vi "Teleop.vi"(10 "Match Info":T1={"Autonomous Elapsed Seconds"=0.0, "TeleOp Elapsed Seconds"=0.0, "Disabled Elapsed Seconds"=0.0, "Visited Autonomous"=FALSE, "Visited TeleOp"=FALSE, "Visited Disabled"=FALSE, "Autonomous Settings"={"Autonomous Style"=enum."Independent", "VI Refnum"=refnum}}, 11 "Call Context":T2) -> ()   [LabVIEW 2012]
doc: "This VI is called for each TeleOp packet received from the DS where the robot is not disabled. It is often used to read from the joysticks and update I/O or to update setpoints for timed control loops. It should complete and return within 20 milliseconds or it may miss DS packets."
uses:
  <vilib>/Rock Robotics/WPI/DriverStation/WPI_DriverStationDerivedRobotMode.ctl
  <vilib>/Rock Robotics/WPI/DriverStation/WPI_DriverStationMatch Info.ctl
  RefnameEnum.ctl
  QueueEnum.ctl
  Robot Global Data.vi
  <vilib>/Rock Robotics/WPI/Joystick/WPI_JoystickGetSetRefNum.vi
  State_Machine_Enum.ctl
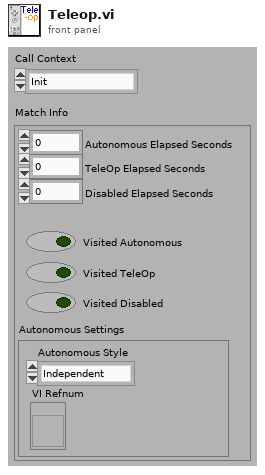
[diagram p1: front panel]
types:
  T1 = typedef "WPI_DriverStationMatch Info.ctl" = cluster{"Autonomous Elapsed Seconds":dbl, "TeleOp Elapsed Seconds":dbl, "Disabled Elapsed Seconds":dbl, "Visited Autonomous":bool, "Visited TeleOp":bool, "Visited Disabled":bool, "Autonomous Settings":cluster{"Autonomous Style":enum16{"Iterative", "Independent"}, "VI Refnum":refnum<vi>}}
  T2 = typedef "WPI_DriverStationDerivedRobotMode.ctl" = enum16{"Init", "Execute", "Stop"}
  T3 = typedef "State_Machine_Enum.ctl" = enum16{"Idle", "Start", "Do", "Stop", "Init"}
  T4 = typedef "QueueEnum.ctl" = enum16{"cTankDrive", "cClimb", "cLauncherAngle", "cLauncherWheel", "cFirePneumatic"}
  T5 = typedef "RefnameEnum.ctl" = enum16{"FireLauncher", "Climber", "Shield", "TankDrive", "DriveEncoderL", "DriveEncoderR", "LauncherMotorRPM", "LauncherEncoderAnalog", "LauncherEncoderRPM", "ShooterLS", "DriveAlignLSLeft", "DriveAlignLSRight", "ClimbingLS", "LauncherEncoderAngle", "LauncherMotorAngle", "Gamepad1", "Gamepad2", "Compressor", "ClimbWeightSol3", "ClimbWeightSol4"}
  T6 = typedef "WPI_JoystickDevRef.ctl" = cluster{"Device":T7}
  T7 = typedef "WPI_JoystickDeviceEnum.ctl" = enum16{"USB 1", "USB 2", "USB 3", "USB 4", "Kinect 1", "Kinect 2"}
  T8 = typedef "WPI_JoystickButtonState.ctl" = cluster{"Button 1":bool, "Button 2":bool, "Button 3":bool, "Button 4":bool, "Button 5":bool, "Button 6":bool, "Button 7":bool, "Button 8":bool, "Button 9":bool, "Button 10":bool, "Button 11":bool, "Button 12":bool}
  T9 = cluster{"axis 1 (x)":dbl, "axis 2 (y)":dbl, "axis 3 (throttle)":dbl, "axis 4":dbl, "axis 5":dbl, "axis 6":dbl}
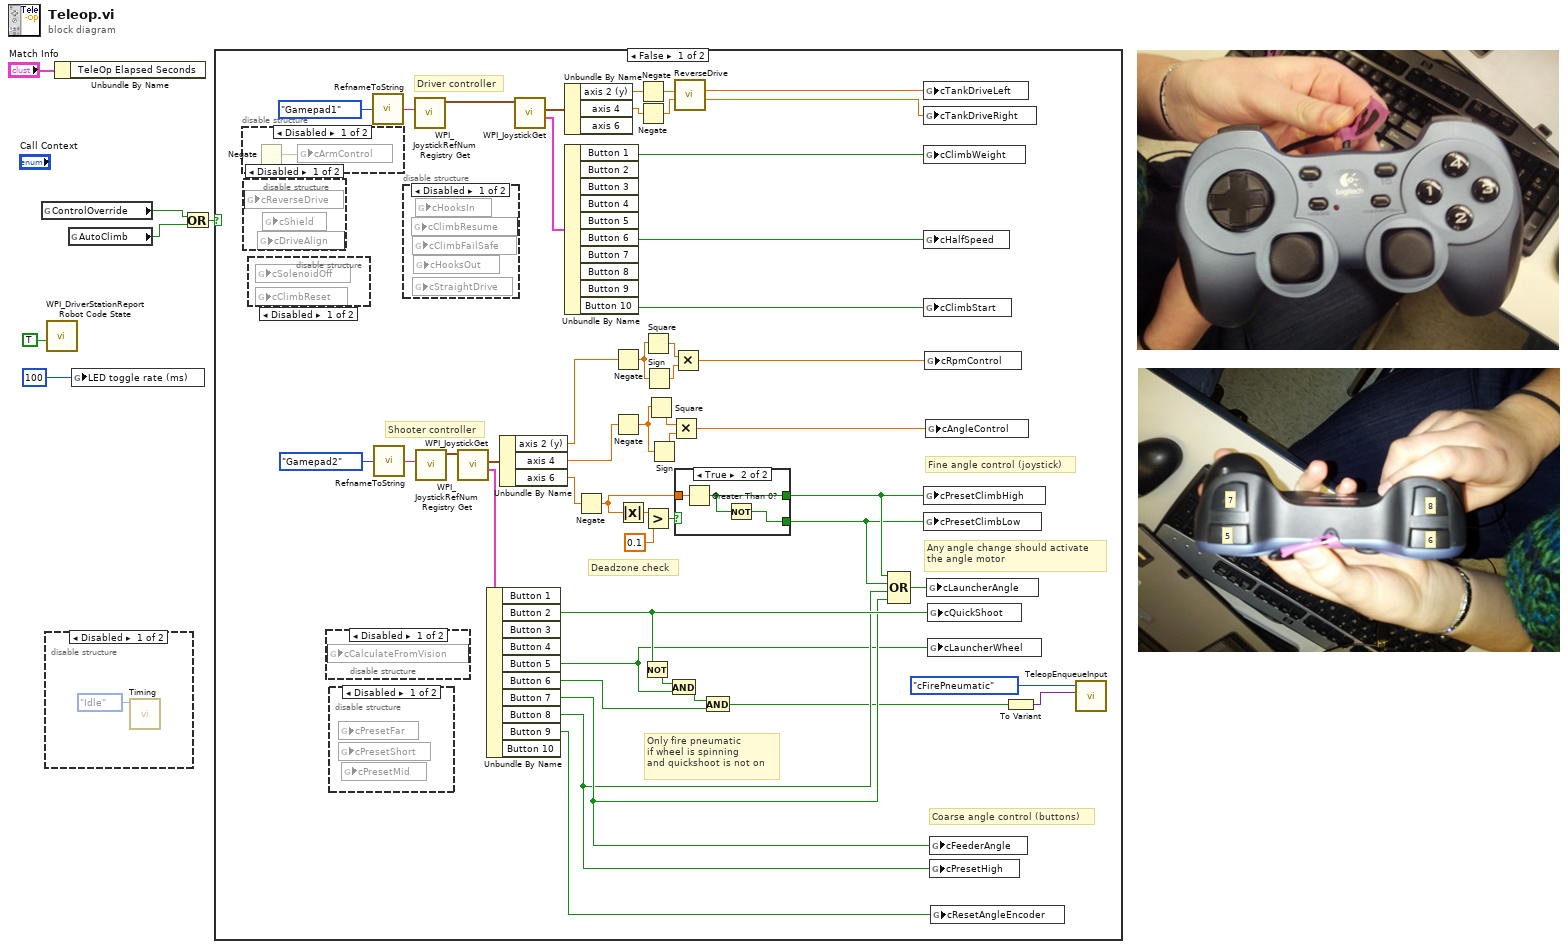
[diagram p0: block diagram]
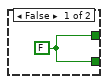
[diagram p5: hidden frame]
diagram:
  # "5"
  # "7"
  # "6"
  # "8"
  n1 = global read "Robot Global Data.vi" "ControlOverride"() -> (w3:bool)
  n2 = disable-structure shown="Disabled" {
    frame Disabled {
      n3 = call "Timing.vi"("State"=State_Machine_Enum."Idle") -> ()  [unwired: 9 in, 2 out]
    }
    frame Enabled {
    }
  }
  n4 = call <vilib>:"WPI_DriverStationReport Robot Code State.vi"("TeleOp"=TRUE ("Autonomous")) -> ()  [unwired: 10 in, 1 out]
  n5 = Unbundle By Name("Match Info") -> ()  [unwired: 1 out]
  n6 = global read "Robot Global Data.vi" "AutoClimb"() -> (w1:bool)
  n7 = global write "Robot Global Data.vi" "LED toggle rate (ms)"(u32 100 ("LED ms toggle rate")) -> ()
  n8 = Or(x=w3, y=w1) -> (x .or. y?=w2:bool)
  n9 = case shown="False" w2 {
    frame False {
      # "Fine angle control (joystick)"
      # "Coarse angle control (buttons)"
      # "Only fire pneumatic\nif wheel is spinning\nand quickshoot is not on"
      # "Deadzone check"
      # "Any angle change should activate\nthe angle motor"
      # "Shooter controller"
      # "Driver controller"
      n10 = disable-structure shown="Disabled" {
        frame Disabled {
          n11 = Negate() -> (-x=w60:dbl)  [unwired: 1 in]
          n12 = global write "Robot Global Data.vi" "cArmControl"(w60) -> ()
        }
        frame Enabled {
        }
      }
      n13 = disable-structure shown="Disabled" {
        frame Disabled {
          n14 = global read "Robot Global Data.vi" "cReverseDrive"() -> ()  [unwired: 1 in]
          n15 = global read "Robot Global Data.vi" "cDriveAlign"() -> ()  [unwired: 1 in]
          n16 = global read "Robot Global Data.vi" "cShield"() -> ()  [unwired: 1 in]
        }
        frame Enabled {
        }
      }
      n17 = disable-structure shown="Disabled" {
        frame Disabled {
          n18 = global read "Robot Global Data.vi" "cSolenoidOff"() -> ()  [unwired: 1 in]
          n19 = global read "Robot Global Data.vi" "cClimbReset"() -> ()  [unwired: 1 in]
        }
        frame Enabled {
        }
      }
      n20 = disable-structure shown="Disabled" {
        frame Disabled {
          n21 = global read "Robot Global Data.vi" "cCalculateFromVision"() -> ()  [unwired: 1 in]
        }
        frame Enabled {
        }
      }
      n22 = disable-structure shown="Disabled" {
        frame Disabled {
          n23 = global read "Robot Global Data.vi" "cPresetFar"() -> ()  [unwired: 1 in]
          n24 = global read "Robot Global Data.vi" "cPresetShort"() -> ()  [unwired: 1 in]
          n25 = global read "Robot Global Data.vi" "cPresetMid"() -> ()  [unwired: 1 in]
        }
        frame Enabled {
        }
      }
      n26 = call "RefnameToString.vi"("Enum"=RefnameEnum."Gamepad1") -> ("Refname"=w30:string)
      n27 = call "RefnameToString.vi"("Enum"=RefnameEnum."Gamepad2") -> ("Refname"=w28:string)
      n28 = disable-structure shown="Disabled" {
        frame Disabled {
          n29 = global read "Robot Global Data.vi" "cClimbResume"() -> ()  [unwired: 1 in]
          n30 = global read "Robot Global Data.vi" "cClimbFailSafe"() -> ()  [unwired: 1 in]
          n31 = global read "Robot Global Data.vi" "cStraightDrive"() -> ()  [unwired: 1 in]
          n32 = global read "Robot Global Data.vi" "cHooksOut"() -> ()  [unwired: 1 in]
          n33 = global read "Robot Global Data.vi" "cHooksIn"() -> ()  [unwired: 1 in]
        }
        frame Enabled {
        }
      }
      n34 = call <vilib>:"WPI_JoystickRefNum Registry Get.vi"("refnum name"=w30) -> ("JoystickDevRef"=w55:T6)  [unwired: 1 in, 9 out]
      n35 = call <vilib>:"WPI_JoystickRefNum Registry Get.vi"("refnum name"=w28) -> ("JoystickDevRef"=w54:T6)  [unwired: 1 in, 9 out]
      n36 = call <vilib>:"WPI_JoystickGet.vi"("JoystickDevRef"=w54) -> ("Buttons"=w49:T8, "Axes"=w50:T9)  [unwired: 4 in, 1 out]
      n37 = Unbundle By Name(w49) -> ("Button 2"=w21:bool, "Button 5"=w13:bool, "Button 6"=w12:bool, "Button 7"=w16:bool, "Button 8"=w15:bool, "Button 9"=w32:bool)  [unwired: 4 out]
      n38 = Unbundle By Name(w50) -> ("axis 2 (y)"=w47:dbl, "axis 4"=w45:dbl, "axis 6"=w27:dbl)
      n39 = call <vilib>:"WPI_JoystickGet.vi"("JoystickDevRef"=w55) -> ("Buttons"=w51:T8, "Axes"=w53:T9)  [unwired: 4 in, 1 out]
      n40 = Unbundle By Name(w53) -> ("axis 2 (y)"=w52:dbl, "axis 4"=w36:dbl)  [unwired: 1 out]
      n41 = Unbundle By Name(w51) -> ("Button 1"=w23:bool, "Button 6"=w42:bool, "Button 10"=w43:bool)  [unwired: 7 out]
      n42 = Negate(x=w27) -> (-x=w22:dbl)
      n43 = Negate(x=w47) -> (-x=w39:dbl)
      n44 = Negate(x=w45) -> (-x=w38:dbl)
      n45 = Absolute Value(x=w22) -> (abs(x)=w26:dbl)
      n46 = Negate(x=w52) -> (-x=w37:dbl)
      n47 = Negate(x=w36) -> (-x=w35:dbl)
      n48 = Not(x=w21) -> (.not. x?=w14:bool)
      n49 = Square(x=w39) -> (x^2=w48:dbl)
      n50 = Greater?(x=w26, y=0.1) -> (0:w25:bool)
      n51 = Sign(1:w39) -> (0:w17:dbl)
      n52 = Square(x=w38) -> (x^2=w44:dbl)
      n53 = Sign(1:w38) -> (0:w46:dbl)
      n54 = And(x=w14, y=w13) -> (x .and. y?=w10:bool)
      n55 = Multiply(x=w44, y=w46) -> (x*y=w40:dbl)
      n56 = Multiply(x=w48, y=w17) -> (x*y=w41:dbl)
      n57 = call "ReverseDrive.vi"("InitLeft"=w37, "InitRight"=w35) -> ("Final Left"=w34:dbl, "FinalRight"=w33:dbl)  [unwired: 7 in]
      n58 = case shown="True" w25 {
        tunnel: w22 -> [_ w59]
        tunnel: [w56 w58] -> w20
        tunnel: [w56 w57] -> w19
        frame False {
          w56 = FALSE
        }
        frame True {
          n59 = Greater Than 0?(x=w59) -> (x > 0?=w58:bool)
          n60 = Not(x=w58) -> (.not. x?=w57:bool)
        }
      }
      n61 = And(x=w10, y=w12) -> (x .and. y?=w11:bool)
      n62 = Compound Arithmetic op=OR(w20, w19, w15, w16) -> (w18:bool)
      n63 = global write "Robot Global Data.vi" "cTankDriveLeft"(w34) -> ()
      n64 = global write "Robot Global Data.vi" "cTankDriveRight"(w33) -> ()
      n65 = global write "Robot Global Data.vi" "cClimbWeight"(w23) -> ()
      n66 = global write "Robot Global Data.vi" "cHalfSpeed"(w42) -> ()
      n67 = global write "Robot Global Data.vi" "cClimbStart"(w43) -> ()
      n68 = global write "Robot Global Data.vi" "cPresetClimbHigh"(w20) -> ()
      n69 = global write "Robot Global Data.vi" "cPresetClimbLow"(w19) -> ()
      n70 = global write "Robot Global Data.vi" "cRpmControl"(w41) -> ()
      n71 = global write "Robot Global Data.vi" "cAngleControl"(w40) -> ()
      n72 = global write "Robot Global Data.vi" "cLauncherAngle"(w18) -> ()
      n73 = global write "Robot Global Data.vi" "cQuickShoot"(w21) -> ()
      n74 = global write "Robot Global Data.vi" "cLauncherWheel"(w13) -> ()
      n75 = global write "Robot Global Data.vi" "cFeederAngle"(w16) -> ()
      n76 = global write "Robot Global Data.vi" "cPresetHigh"(w15) -> ()
      n77 = global write "Robot Global Data.vi" "cResetAngleEncoder"(w32) -> ()
      n78 = To Variant(anything=w11) -> (Variant=w8:variant)
      n79 = call "TeleopEnqueueInput.vi"("Variant"=w8, "QueueEnum"=QueueEnum."cFirePneumatic" ("Queue")) -> ()  [unwired: 9 in, 1 out]
    }
    frame True {
    }
  }
